vi "(SubVI) Initiate Image Buffer.vi"(11 "Image Type":T2 items=["Grayscale (U8)", "Grayscale (I16)", "Grayscale (SGL)", "Complex (CSG)", "RGB (U32)", "HSL (U32)", "RGB (U64)", "Grayscale (U16)"]) -> (2 "# Of Buffers":i32, 3 "Image Buffer":T1[](array[typedef]))   [LabVIEW 2014]
uses:
  <vilib>/vision/Image Controls.llb/IMAQ Image.ctl
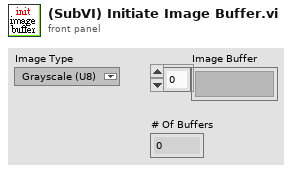
[diagram p1: front panel]
types:
  T1 = typedef "IMAQ Image.ctl" = refnum<image>
  T2 = typedef "Image Type" = u32
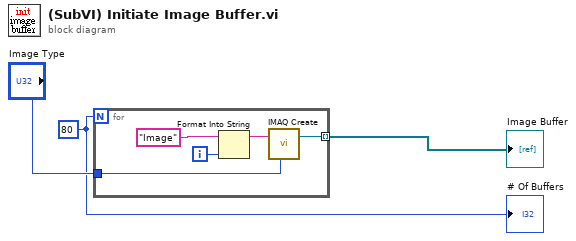
[diagram p0: block diagram]
diagram:
  w2 = 80 ("# Of Buffers")
  n1 = for {
    N: w2 -> [_]
    tunnel: [w8] -> w1 mode=indexing
    tunnel: "Image Type" -> [w4]
    i -> [w7]
    n2 = Format Into String(initial string="Image" ("Image Name"), w7) -> (resulting string=w5:string)  [unwired: 2 in, 1 out]
    n3 = call "IMAQ Create"("Image Name"=w5, "Image Type"=w4) -> ("New Image"=w8:T1)  [unwired: 3 in, 1 out]
  }
  "Image Buffer" <- w1
  "# Of Buffers" <- w2
